vi "关闭所有串口.vi"   [LabVIEW 2017]
uses:
  <vilib>/Instr/_visa.llb/VISA Find Search Mode.ctl
types:
  T1 = typedef "VISA Find Search Mode.ctl" = u32
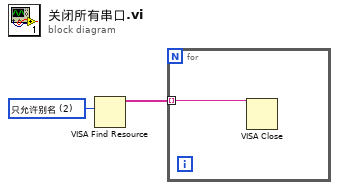
[diagram p0: block diagram]
diagram:
  w2 = T1 2 items=["仅允许规范名称"=0, "只允许别名"=2, "包含匹配别名"=3, "包含所有别名"=4] ("Search Mode")
  n1 = VISA Find Resource(10:w2) -> (3:w1:string[])  [unwired: 2 in, 2 out]
  n2 = for {
    tunnel: w1 -> [w3] mode=indexing
    n3 = VISA Close(VISA resource name=w3) -> ()  [unwired: 1 in, 1 out]
  }
